vi "Add Widget to Container.vi"(5 "Container":refnum<class "QWidget.lvclass">, 8 "Error In":errorcluster, 9 "Label":string, 10 "Widget":refnum<class "QWidget.lvclass">, 11 "Tab Widget Builder in":refnum<class "Tab Widget Builder.lvclass">) -> (0 "Error Out":errorcluster, 3 "Tab Widget Builder out":refnum<class "Tab Widget Builder.lvclass">)   [LabVIEW 2014, in "Tab Widget Builder.lvclass"]
doc: "Implements the interface provided by Abstract Widget Builder.\n\n\nCopyright (c) 2019 Sze Howe Koh.\nThis code is licensed under the MIT license."
uses:
  Tab Widget Builder.lvclass
  <vilib>/addons/LQ/Qt Widgets/QWidget/QWidget.lvclass
  <vilib>/addons/LQ/Qt Widgets/QTabWidget/QTabWidget.lvclass
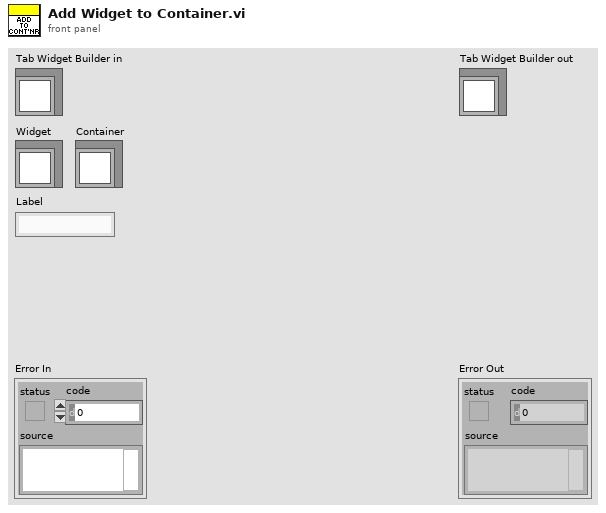
[diagram p1: front panel]
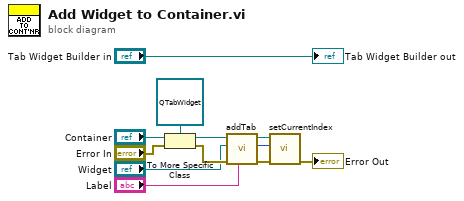
[diagram p0: block diagram]
diagram:
  n1 = To More Specific Class(target class=refnum<class "QTabWidget.lvclass"> refnum ("QTabWidget"), reference="Container", error in="Error In") -> (specific class reference=w9:refnum<class "QTabWidget.lvclass">, error out=w7:errorcluster)
  n2 = call <vilib>:"addTab.vi"("label"="Label", "Error In"=w7, "widget"="Widget", "QTabWidget In"=w9) -> ("Error Out"=w3:errorcluster, "Value"=w1:i32, "QTabWidget Out"=w2:refnum<class "QTabWidget.lvclass">)  [unwired: 5 in]
  n3 = call <vilib>:"setCurrentIndex.vi"("Error In"=w3, "index"=w1, "QTabWidget In"=w2) -> ("Error Out"=→"Error Out":errorcluster)  [unwired: 7 in, 1 out]
  "Tab Widget Builder out" <- "Tab Widget Builder in"
